vi "Init.vi"(8 "error in (no error)":errorcluster, 11 "UI Actor in":refnum<class "UI Actor.lvclass">) -> (0 "error out":errorcluster, 3 "UI Actor out":refnum<class "UI Actor.lvclass">)   [LabVIEW 2020, in "UI Actor.lvlib" / "UI Actor.lvclass"]
uses:
  UI Actor.lvclass
  C:/Program Files (x86)/National Instruments/LabVIEW 2020/vi.lib/ActorFramework/Actor/Actor.lvclass
  MSG/MSG.lvclass
  UI Actor.lvclass/UI Actor.ctl
  Cafe/Cafe.lvclass
  Cafe/Cafe.lvclass/Cafe.ctl
  Coca/Coca.lvclass
  Coca/Coca.lvclass/Coca.ctl
  USD Actor/USD Actor.lvclass
  USD Actor/USD Actor.lvclass/USD Actor.ctl
  MXN Actor/MXN Actor.lvclass
  MXN Actor/MXN Actor.lvclass/MXN Actor.ctl
  MSG/MSG.lvclass/MSG.ctl
  MSG Messages/Update MSG Msg/Update MSG Msg.lvclass/Update MSG Msg.ctl
  <vilib>/ActorFramework/Message Enqueuer/Message Enqueuer.lvclass/Message Enqueuer.ctl
  Cafe/Write Sub Panel Products.vi
  Cafe/Write MXN.vi
  Cafe/Write Idioma.vi
  Coca/Write Sub Panel Products.vi
  Coca/Write MXN.vi
  Coca/Write Idioma.vi
  Read Idioma.vi
  <vilib>/ActorFramework/Message Enqueuer/Enqueue.vi
  MSG Messages/Update MSG Msg/Update MSG Msg.lvclass
  C:/Program Files (x86)/National Instruments/LabVIEW 2020/vi.lib/ActorFramework/Message/Message.lvclass
  <vilib>/ActorFramework/Message Priority Queue/Priority Enqueue.vi
  <vilib>/ActorFramework/Actor/Actor.lvclass
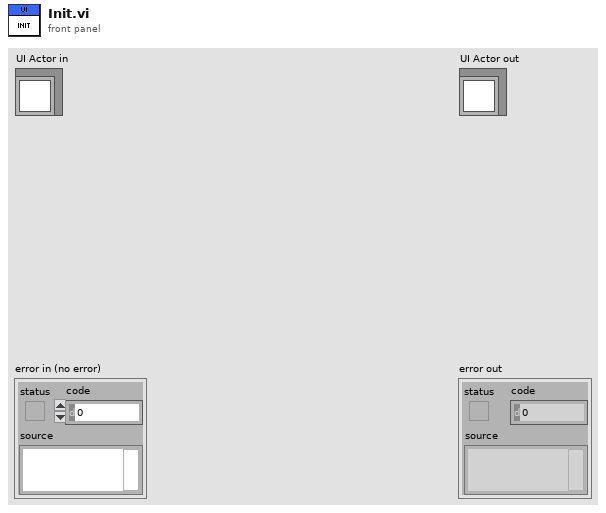
[diagram p1: front panel]
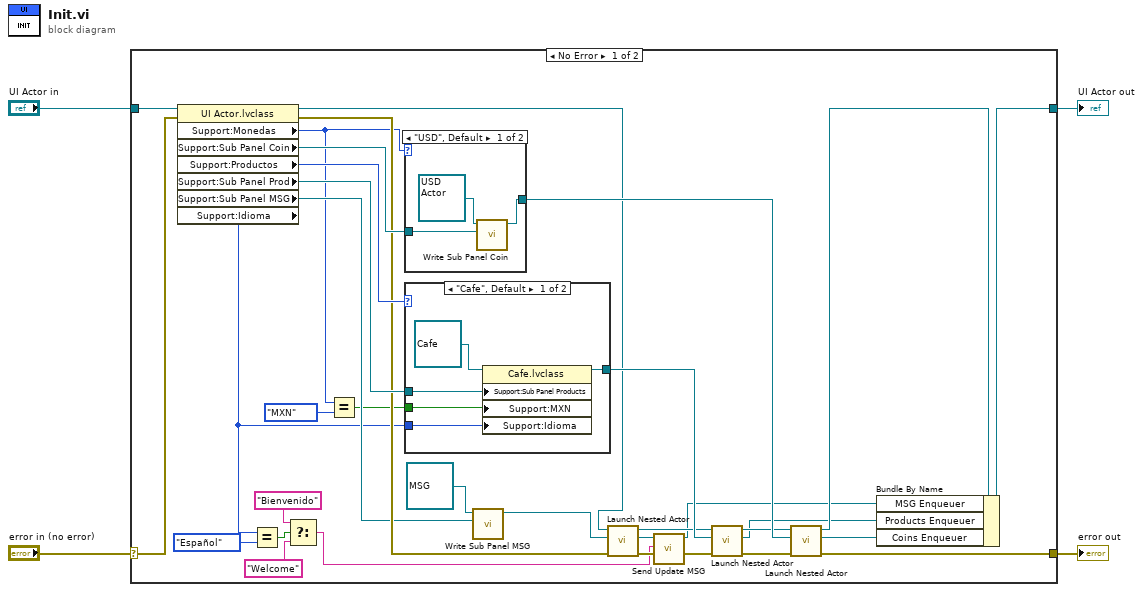
[diagram p0: block diagram]
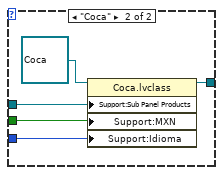
[diagram p2: hidden frame]
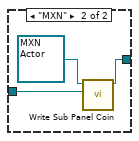
[diagram p3: hidden frame]
diagram:
  n1 = case shown="No Error" "error in (no error)" {
    selector: "error in (no error)" -> [w36 w55]
    tunnel: [w35 w55] -> w3
    tunnel: [w33 w54] -> w1
    tunnel: "UI Actor in" -> [w37 w54]
    frame No Error {
      n2 = property class="UI Actor.lvclass"(reference=w37, error in=w36) -> (reference out=w22:refnum<class "UI Actor.lvclass">, error out=w23:errorcluster, "Support:Monedas"=w16:enum16{"USD", "MXN"}, "Support:Sub Panel Coin"=w31:refnum<vi>, "Support:Productos"=w30:enum16{"Cafe", "Coca"}, "Support:Sub Panel Prod"=w29:refnum<vi>, "Support:Sub Panel MSG"=w18:refnum<vi>, "Support:Idioma"=w5:enum16{"Español", "Ingles"})
      n3 = Equal?(x=w5, y=enum16{"Español", "Ingles"}."Español") -> (x = y?=w14:bool)
      n4 = Select(t="Bienvenido", s=w14, f="Welcome") -> (s? t:f=w6:string)
      n5 = Equal?(x=w16, y=enum16{"USD", "MXN"}."MXN") -> (x = y?=w17:bool)
      n6 = case shown="\"USD\", Default" w16 {
        tunnel: w31 -> [w50 w53]
        tunnel: [w48 w51] -> w28
        frame "USD", Default {
          n7 = call "Write Sub Panel Coin.vi"("Sub Panel Coin"=w50, "USD Actor in"=refnum<class "USD Actor.lvclass"> refnum ("USD Actor.lvlib:USD Actor.lvclass")) -> ("USD Actor out"=w48:refnum<class "USD Actor.lvclass">)  [unwired: 8 in, 1 out]
        }
        frame "MXN" {
          n8 = call "Write Sub Panel Coin.vi"("Sub Panel Coin"=w53, "MXN Actor in"=refnum<class "MXN Actor.lvclass"> refnum ("MXN Actor.lvlib:MXN Actor.lvclass")) -> ("MXN Actor out"=w51:refnum<class "MXN Actor.lvclass">)  [unwired: 8 in, 1 out]
        }
      }
      n9 = case shown="\"Cafe\", Default" w30 {
        tunnel: w29 -> [w40 w45]
        tunnel: [w41 w46] -> w25
        tunnel: w17 -> [w39 w44]
        tunnel: w5 -> [w38 w43]
        frame "Cafe", Default {
          n10 = property class="Cafe.lvclass"(reference=refnum<class "Cafe.lvclass"> refnum ("Cafe.lvlib:Cafe.lvclass"), "Support:Sub Panel Products"=w40, "Support:MXN"=w39, "Support:Idioma"=w38) -> (reference out=w41:refnum<class "Cafe.lvclass">)  [unwired: 1 in, 1 out]
        }
        frame "Coca" {
          n11 = property class="Coca.lvclass"(reference=refnum<class "Coca.lvclass"> refnum ("Coca.lvlib:Coca.lvclass"), "Support:Sub Panel Products"=w45, "Support:MXN"=w44, "Support:Idioma"=w43) -> (reference out=w46:refnum<class "Coca.lvclass">)  [unwired: 1 in, 1 out]
        }
      }
      n12 = call "Write Sub Panel MSG.vi"("Sub Panel MSG"=w18, "MSG in"=refnum<class "MSG.lvclass"> refnum ("MSG.lvlib:MSG.lvclass")) -> ("MSG out"=w19:refnum<class "MSG.lvclass">)  [unwired: 8 in, 1 out]
      n13 = call <vilib>:"Launch Nested Actor.vi"("error in (no error)"=w23, "Nested Actor"=w19, "Caller Actor in"=w22) -> ("error out"=w8:errorcluster, "Nested Actor's Enqueuer"=w10:refnum<class "Message Enqueuer.lvclass">, "Caller Actor out"=w21:refnum<class "UI Actor.lvclass">)  [unwired: 6 in]
      n14 = call "Send Update MSG.vi"("error in (no error)"=w8, "MSG"=w6, "Message Enqueuer"=w10) -> ("error out"=w7:errorcluster, "Message Enqueuer out"=w9:refnum<class "Message Enqueuer.lvclass">)  [unwired: 7 in]
      n15 = call <vilib>:"Launch Nested Actor.vi"("error in (no error)"=w7, "Nested Actor"=w25, "Caller Actor in"=w21) -> ("error out"=w27:errorcluster, "Nested Actor's Enqueuer"=w24:refnum<class "Message Enqueuer.lvclass">, "Caller Actor out"=w26:refnum<class "UI Actor.lvclass">)  [unwired: 6 in]
      n16 = call <vilib>:"Launch Nested Actor.vi"("error in (no error)"=w27, "Nested Actor"=w28, "Caller Actor in"=w26) -> ("error out"=w35:errorcluster, "Nested Actor's Enqueuer"=w32:refnum<class "Message Enqueuer.lvclass">, "Caller Actor out"=w34:refnum<class "UI Actor.lvclass">)  [unwired: 6 in]
      n17 = Bundle By Name(cluster=w34, "MSG Enqueuer"=w9, "Products Enqueuer"=w24, "Coins Enqueuer"=w32) -> (w33:refnum<class "UI Actor.lvclass">)
    }
    frame Error {
    }
  }
  "error out" <- w3
  "UI Actor out" <- w1
